vi "proj_dzialanie_na_planszy.vi"(6 "Table control":refnum<vi>, 9 "Tabela sprawdzajaca":refnum<vi>, 10 "Plansza gry":refnum<vi>, 11 "Table in":refnum<vi>) -> (1 "Przegrana":bool, 2 "Plansza sprawdzajaca":i32[][](array[numeric]), 3 "Ilosc min dookola pola":i32, 4 "Reset gry":bool, 5 "Wygrana":bool)   [LabVIEW 2020]
uses:
  <vilib>/Utility/miscctls.llb/LVRowAndColumnTypeDef.ctl
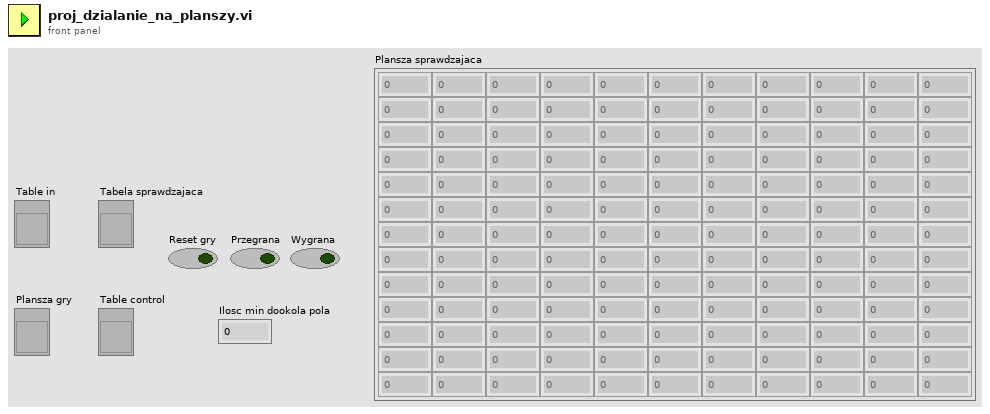
[diagram p1: front panel]
types:
  T1 = typedef "LVRowAndColumnTypeDef.ctl" = cluster{"Row":i32, "Column":i32}
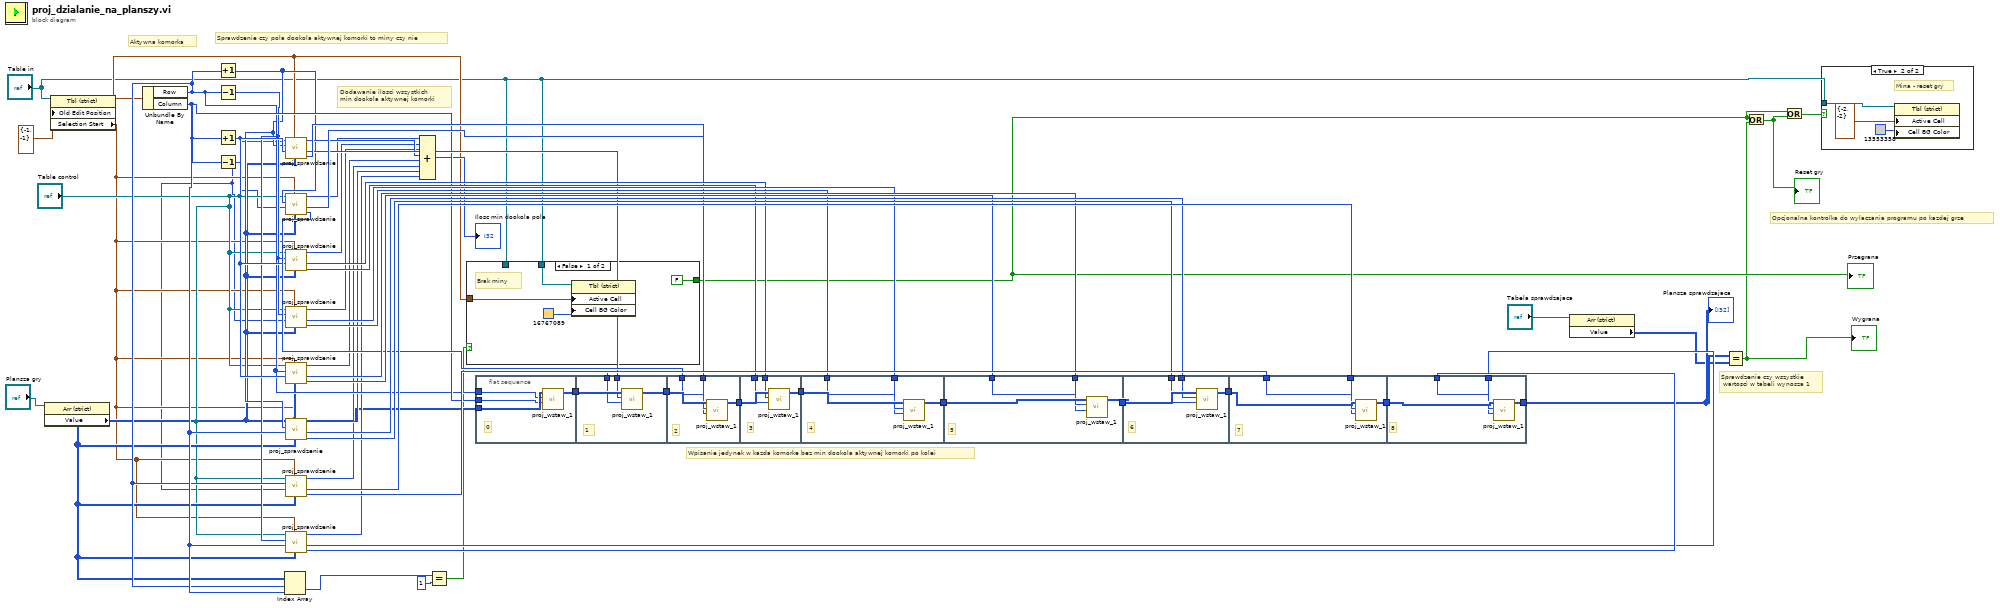
[diagram p0: block diagram]
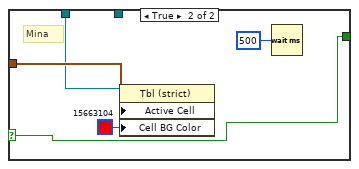
[diagram p3: hidden frame]
diagram:
  # "Sprawdzenie czy pola dookola aktywnej komorki to miny czy nie"
  # "Dodawanie ilosci wszystkich \nmin dookola aktywnej komorki"
  # "Sprawdzenie czy wszystkie\n wartosci w tabeli wynosza 1"
  # "Opcjonalna kontrolka do wylaczania programu po kazdej grze"
  # "Aktywna komorka"
  # "Wpisanie jedynek w kazda komorke bez min dookola aktywnej komorki po kolei"
  n1 = property class="Arr (strict)"(reference="Plansza gry") -> ("Value"=w17:i32[][])  [unwired: 1 in, 2 out]
  n2 = property on="Property Node" class="Tbl (strict)"(reference="Table in", "Old Edit Position"=cluster{"Row":i32, "Column":i32} {"Row"=-1, "Column"=-1} ("Edit Position")) -> ("Selection Start"=w15:T1)  [unwired: 1 in, 2 out]
  n3 = Unbundle By Name(w15) -> ("Row"=w29:i32, "Column"=w30:i32)
  n4 = Increment(x=w29) -> (x+1=w18:i32)
  n5 = Decrement(x=w29) -> (x-1=w19:i32)
  n6 = Increment(x=w30) -> (x+1=w33:i32)
  n7 = Decrement(x=w30) -> (x-1=w14:i32)
  n8 = Index Array(array=w17, index (row)=w29, index (col)=w30) -> (element=w6:i32)
  n9 = call "proj_sprawdzenie.vi"("Plansza"=w17, "Selection Start"=w15, "Kolumna"=w33, "Wiersz"=w18, "Tabela interaktywna"="Table control") -> ("Kolumna wychodzaca"=w32:i32, "Wiersz wychodzacy"=w31:i32, "Numeric"=w23:i32)  [unwired: 4 in]
  n10 = call "proj_sprawdzenie.vi"("Plansza"=w17, "Selection Start"=w15, "Kolumna"=w14, "Wiersz"=w18, "Tabela interaktywna"="Table control") -> ("Kolumna wychodzaca"=w35:i32, "Wiersz wychodzacy"=w34:i32, "Numeric"=w20:i32)  [unwired: 4 in]
  n11 = call "proj_sprawdzenie.vi"("Plansza"=w17, "Selection Start"=w15, "Kolumna"=w33, "Wiersz"=w19, "Tabela interaktywna"="Table control") -> ("Kolumna wychodzaca"=w37:i32, "Wiersz wychodzacy"=w36:i32, "Numeric"=w21:i32)  [unwired: 4 in]
  n12 = call "proj_sprawdzenie.vi"("Plansza"=w17, "Selection Start"=w15, "Kolumna"=w14, "Wiersz"=w19, "Tabela interaktywna"="Table control") -> ("Kolumna wychodzaca"=w39:i32, "Wiersz wychodzacy"=w38:i32, "Numeric"=w22:i32)  [unwired: 4 in]
  n13 = call "proj_sprawdzenie.vi"("Plansza"=w17, "Selection Start"=w15, "Kolumna"=w33, "Wiersz"=w29, "Tabela interaktywna"="Table control") -> ("Kolumna wychodzaca"=w41:i32, "Wiersz wychodzacy"=w40:i32, "Numeric"=w24:i32)  [unwired: 4 in]
  n14 = call "proj_sprawdzenie.vi"("Plansza"=w17, "Selection Start"=w15, "Kolumna"=w30, "Wiersz"=w18, "Tabela interaktywna"="Table control") -> ("Kolumna wychodzaca"=w43:i32, "Wiersz wychodzacy"=w42:i32, "Numeric"=w26:i32)  [unwired: 4 in]
  n15 = call "proj_sprawdzenie.vi"("Plansza"=w17, "Selection Start"=w15, "Kolumna"=w14, "Wiersz"=w29, "Tabela interaktywna"="Table control") -> ("Kolumna wychodzaca"=w45:i32, "Wiersz wychodzacy"=w44:i32, "Numeric"=w25:i32)  [unwired: 4 in]
  n16 = call "proj_sprawdzenie.vi"("Plansza"=w17, "Selection Start"=w15, "Kolumna"=w30, "Wiersz"=w19, "Tabela interaktywna"="Table control") -> ("Kolumna wychodzaca"=w47:i32, "Wiersz wychodzacy"=w46:i32, "Numeric"=w27:i32)  [unwired: 4 in]
  n17 = Compound Arithmetic op=ADD(w20, w21, w22, w23, w24, w25, w26, w27) -> (→"Ilosc min dookola pola":i32)
  n18 = Equal?(x=w6, y=1) -> (x = y?=w11:bool)
  n19 = case shown="False" w11 {
    selector: w11 -> [_ w63]
    tunnel: w15 -> [w58 w62]
    tunnel: [FALSE w63] -> w13
    tunnel: "Table in" -> [w56 _]
    tunnel: "Table in" -> [_ w60]
    frame False {
      # "Brak miny"
      n20 = property on="Property Node" class="Tbl (strict)"(reference=w56, "Active Cell"=w58, "Cell BG Color"=u32 16767089 ("Active Cell:Cell Background Color")) -> ()  [unwired: 1 in, 2 out]
    }
    frame True {
      # "Mina"
      n21 = property on="Property Node" class="Tbl (strict)"(reference=w60, "Active Cell"=w62, "Cell BG Color"=u32 15663104 ("Active Cell:Cell Background Color")) -> ()  [unwired: 1 in, 2 out]
      n22 = Wait (ms)(milliseconds to wait=u32 500) -> ()  [unwired: 1 out]
    }
  }
  "Przegrana" <- w13
  n23 = flat-sequence {
    tunnel: w17 -> [w67]
    tunnel: w29 -> [w66]
    tunnel: w30 -> [w65]
    tunnel: [w68] -> w55
    tunnel: w55 -> [w72]
    tunnel: [w71] -> w54
    tunnel: w31 -> [w70]
    tunnel: w32 -> [w69]
    tunnel: w54 -> [w76]
    tunnel: [w75] -> w53
    tunnel: w34 -> [w74]
    tunnel: w35 -> [w73]
    tunnel: w53 -> [w80]
    tunnel: [w79] -> w52
    tunnel: w36 -> [w78]
    tunnel: w37 -> [w77]
    tunnel: w52 -> [w84]
    tunnel: [w83] -> w51
    tunnel: w38 -> [w82]
    tunnel: w39 -> [w81]
    tunnel: w51 -> [w88]
    tunnel: [w87] -> w50
    tunnel: w40 -> [w86]
    tunnel: w41 -> [w85]
    tunnel: w50 -> [w92]
    tunnel: [w91] -> w49
    tunnel: w42 -> [w90]
    tunnel: w43 -> [w89]
    tunnel: w49 -> [w96]
    tunnel: [w95] -> w48
    tunnel: w44 -> [w94]
    tunnel: w45 -> [w93]
    tunnel: [w99] -> w8
    tunnel: w48 -> [w100]
    tunnel: w46 -> [w98]
    tunnel: w47 -> [w97]
    frame #0 {
      # "0"
      n24 = call "proj_wstaw_1.vi"("Kolumna"=w65, "Wiersz"=w66, "Plansza"=w67) -> ("Plansza sprawdzajaca"=w68:i32[][])  [unwired: 8 in]
    }
    frame #1 {
      # "1"
      n25 = call "proj_wstaw_1.vi"("Kolumna"=w69, "Wiersz"=w70, "Plansza"=w72) -> ("Plansza sprawdzajaca"=w71:i32[][])  [unwired: 8 in]
    }
    frame #2 {
      # "2"
      n26 = call "proj_wstaw_1.vi"("Kolumna"=w73, "Wiersz"=w74, "Plansza"=w76) -> ("Plansza sprawdzajaca"=w75:i32[][])  [unwired: 8 in]
    }
    frame #3 {
      # "3"
      n27 = call "proj_wstaw_1.vi"("Kolumna"=w77, "Wiersz"=w78, "Plansza"=w80) -> ("Plansza sprawdzajaca"=w79:i32[][])  [unwired: 8 in]
    }
    frame #4 {
      # "4"
      n28 = call "proj_wstaw_1.vi"("Kolumna"=w81, "Wiersz"=w82, "Plansza"=w84) -> ("Plansza sprawdzajaca"=w83:i32[][])  [unwired: 8 in]
    }
    frame #5 {
      # "5"
      n29 = call "proj_wstaw_1.vi"("Kolumna"=w85, "Wiersz"=w86, "Plansza"=w88) -> ("Plansza sprawdzajaca"=w87:i32[][])  [unwired: 8 in]
    }
    frame #6 {
      # "6"
      n30 = call "proj_wstaw_1.vi"("Kolumna"=w89, "Wiersz"=w90, "Plansza"=w92) -> ("Plansza sprawdzajaca"=w91:i32[][])  [unwired: 8 in]
    }
    frame #7 {
      # "7"
      n31 = call "proj_wstaw_1.vi"("Kolumna"=w93, "Wiersz"=w94, "Plansza"=w96) -> ("Plansza sprawdzajaca"=w95:i32[][])  [unwired: 8 in]
    }
    frame #8 {
      # "8"
      n32 = call "proj_wstaw_1.vi"("Kolumna"=w97, "Wiersz"=w98, "Plansza"=w100) -> ("Plansza sprawdzajaca"=w99:i32[][])  [unwired: 8 in]
    }
  }
  n33 = property class="Arr (strict)"(reference="Tabela sprawdzajaca") -> ("Value"=w7:i32[][])  [unwired: 1 in, 2 out]
  n34 = Equal?(x=w8, y=w7) -> (x = y?=w12:bool)
  "Wygrana" <- w12
  n35 = Or(x=w13, y=w12) -> (x .or. y?=w9:bool)
  "Reset gry" <- w9
  n36 = Or(x=w13, y=w9) -> (x .or. y?=w10:bool)
  n37 = case shown="True" w10 {
    tunnel: "Table in" -> [_ w101]
    frame False {
      # "Brak miny, nic sie nie dzieje"
    }
    frame True {
      # "Mina - reset gry"
      n38 = property on="Property Node" class="Tbl (strict)"(reference=w101, "Active Cell"=T1 {"Row"=-2, "Column"=-2} ("Active Cell:Active Cell"), "Cell BG Color"=u32 13553358 ("Active Cell:Cell Background Color")) -> ()  [unwired: 1 in, 2 out]
    }
  }
  "Plansza sprawdzajaca" <- w8
